vi "Get Scan Engine Period.vi"(0 "target address (localhost)":string="localhost", 11 "error in (no error)":errorcluster) -> (6 "scan period (uSec)":u32=10000, 15 "error out":errorcluster)   [LabVIEW 2017]
doc: "Returns the scan period of the NI Scan Engine on the target."
uses:
  <resource>/objmgr/ni.var.rc
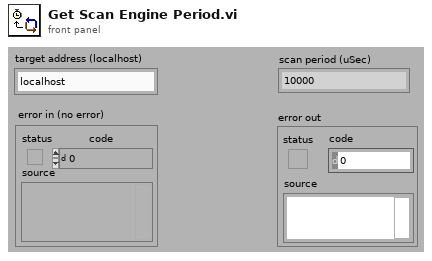
[diagram p1: front panel]
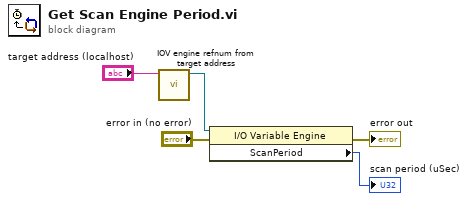
[diagram p0: block diagram]
diagram:
  n1 = call <vilib>:"IOV engine refnum from target address.vi"("target address"="target address (localhost)") -> ("reference out"=w4:refnum<k21>)  [unwired: 10 in]
  n2 = property class="I/O Variable Engine"(reference=w4, error in="error in (no error)") -> (error out=→"error out":errorcluster, "ScanPeriod"=→"scan period (uSec)":u32)  [unwired: 1 out]
